vi "GDSIconEditor_CreateImageMask.vi"(1 "Flood Fill":bool, 2 "8-bit pixmap":u8[][](array[numeric])) -> (0 "Array":u8[](array[numeric]))   [LabVIEW 2020]
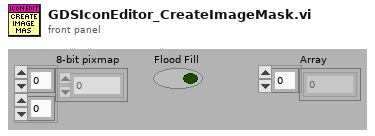
[diagram p1: front panel]
types:
  T1 = cluster{"disabled index (col)":i32, "disabled index (col)":i32}[]
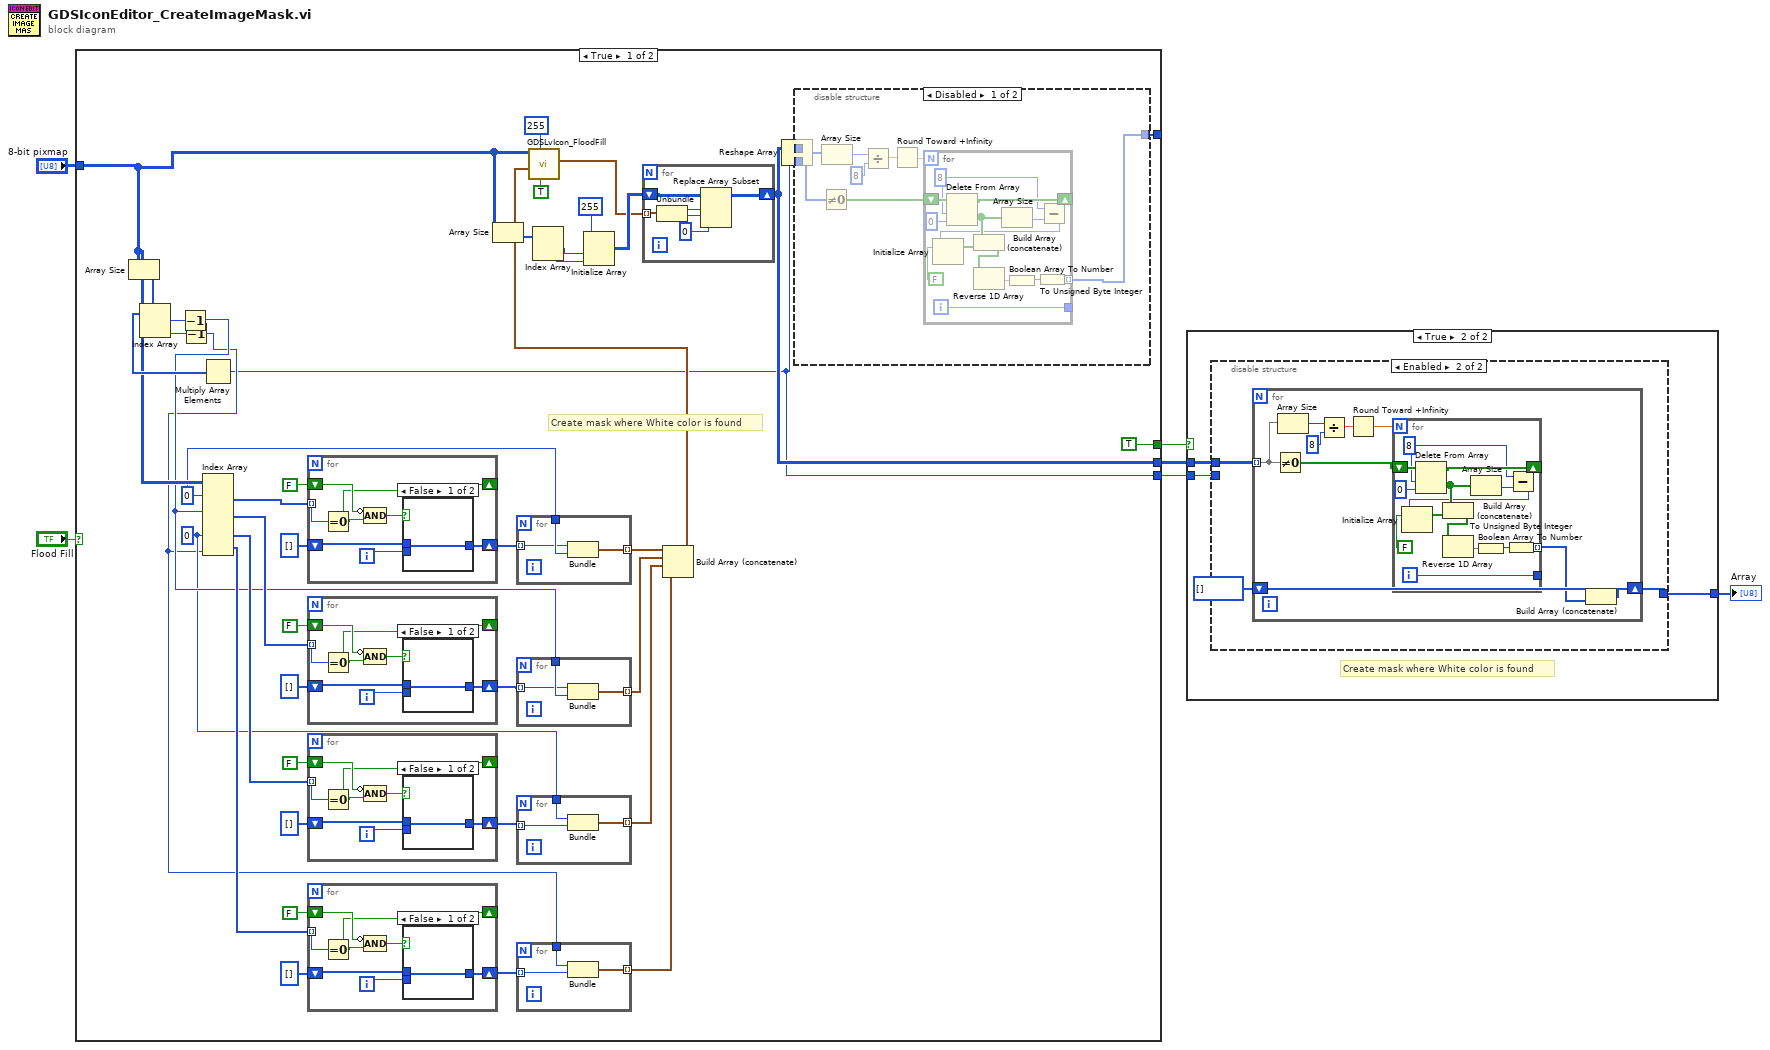
[diagram p0: block diagram]
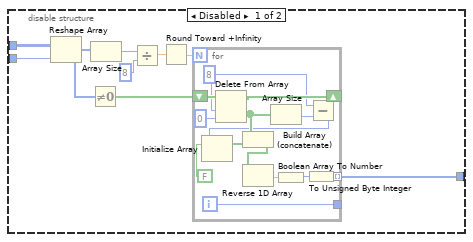
[diagram p3: hidden frame]
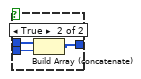
[diagram p5: hidden frame]
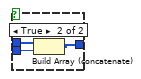
[diagram p6: hidden frame]
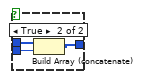
[diagram p7: hidden frame]
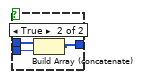
[diagram p8: hidden frame]
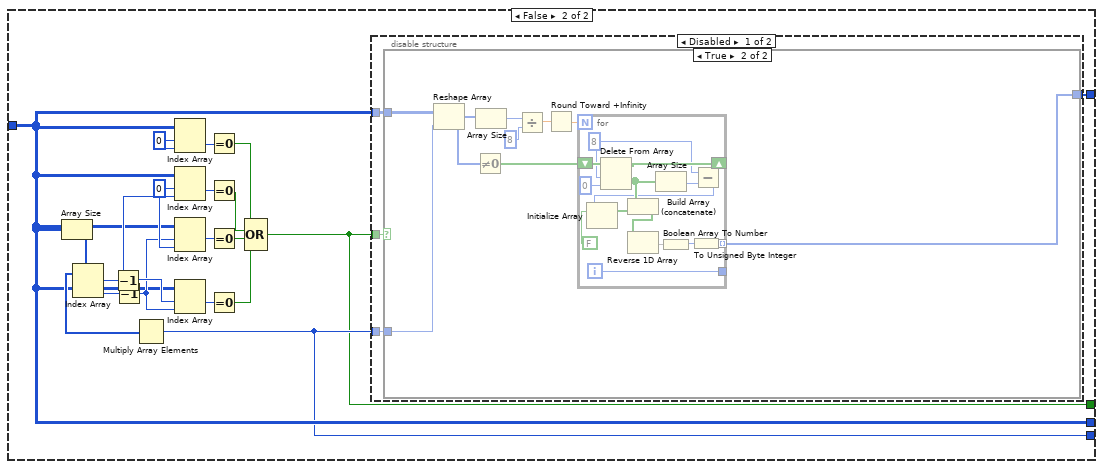
[diagram p9: hidden frame]
diagram:
  n1 = case shown="True" "Flood Fill" {
    tunnel: [w45 w144] -> _
    tunnel: "8-bit pixmap" -> [w43 w135]
    tunnel: [w9 w135] -> w4
    tunnel: [w8 w134] -> w3
    tunnel: [TRUE w133] -> w2
    frame True {
      w29 = 0 ("disabled index (col)")
      w25 = 0 ("disabled index (col)")
      # "Create mask where White color is found"
      n2 = Array Size(array=w43) -> (size(s)=w44:i32[])
      n3 = Index Array(array=w44) -> (element #1=w46:i32, element #2=w47:i32)  [unwired: 2 in]
      n4 = Decrement(x=w46) -> (x-1=w27:i32)
      n5 = Decrement(x=w47) -> (x-1=w23:i32)
      n6 = Multiply Array Elements(1:w44) -> (0:w8:i32)
      n7 = Index Array(array=w43, index (row) #1=w29, index (row) #2=w27, index (col) #3=w25, index (col) #4=w23) -> (element #1=w42:u8[], element #2=w37:u8[], element #3=w32:u8[], element #4=w31:u8[])  [unwired: 4 in]
      n8 = for {
        tunnel: w42 -> [w128] mode=indexing
        shift-right: [w125] -> _
        shift-left: FALSE -> [w127]
        shift-right: [w123] -> w30
        shift-left: i32[] [] -> [w124]
        i -> [w122]
        n9 = Equal To 0?(x=w128) -> (x = 0?=w125:bool)
        n10 = Compound Arithmetic op=AND(invert w127, w125) -> (w126:bool)
        n11 = case shown="False" w126 {
          tunnel: w124 -> [w129 w132]
          tunnel: [w129 w131] -> w123
          tunnel: w122 -> [_ w130]
          frame False {
          }
          frame True {
            n12 = Build Array (concatenate)(w132, w130) -> (w131:i32[])
          }
        }
      }
      n13 = for {
        tunnel: w37 -> [w117] mode=indexing
        shift-right: [w114] -> _
        shift-left: FALSE -> [w116]
        shift-right: [w112] -> w28
        shift-left: i32[] [] -> [w113]
        i -> [w111]
        n14 = Equal To 0?(x=w117) -> (x = 0?=w114:bool)
        n15 = Compound Arithmetic op=AND(invert w116, w114) -> (w115:bool)
        n16 = case shown="False" w115 {
          tunnel: w113 -> [w118 w121]
          tunnel: [w118 w120] -> w112
          tunnel: w111 -> [_ w119]
          frame False {
          }
          frame True {
            n17 = Build Array (concatenate)(w121, w119) -> (w120:i32[])
          }
        }
      }
      n18 = for {
        tunnel: w32 -> [w106] mode=indexing
        shift-right: [w103] -> _
        shift-left: FALSE -> [w105]
        shift-right: [w101] -> w26
        shift-left: i32[] [] -> [w102]
        i -> [w100]
        n19 = Equal To 0?(x=w106) -> (x = 0?=w103:bool)
        n20 = Compound Arithmetic op=AND(invert w105, w103) -> (w104:bool)
        n21 = case shown="False" w104 {
          tunnel: w102 -> [w107 w110]
          tunnel: [w107 w109] -> w101
          tunnel: w100 -> [_ w108]
          frame False {
          }
          frame True {
            n22 = Build Array (concatenate)(w110, w108) -> (w109:i32[])
          }
        }
      }
      n23 = for {
        tunnel: w31 -> [w95] mode=indexing
        shift-right: [w92] -> _
        shift-left: FALSE -> [w94]
        shift-right: [w90] -> w24
        shift-left: i32[] [] -> [w91]
        i -> [w89]
        n24 = Equal To 0?(x=w95) -> (x = 0?=w92:bool)
        n25 = Compound Arithmetic op=AND(invert w94, w92) -> (w93:bool)
        n26 = case shown="False" w93 {
          tunnel: w91 -> [w96 w99]
          tunnel: [w96 w98] -> w90
          tunnel: w89 -> [_ w97]
          frame False {
          }
          frame True {
            n27 = Build Array (concatenate)(w99, w97) -> (w98:i32[])
          }
        }
      }
      n28 = Array Size(array=w43) -> (size(s)=w15:i32[])
      n29 = for {
        tunnel: w30 -> [w87] mode=indexing
        tunnel: w29 -> [w88]
        tunnel: [w86] -> w22 mode=indexing
        n30 = Bundle(w87, "disabled index (col)"=w88) -> (w86:cluster{i32, "disabled index (col)":i32})  [unwired: 1 in]
      }
      n31 = for {
        tunnel: w28 -> [w84] mode=indexing
        tunnel: w27 -> [w85]
        tunnel: [w83] -> w21 mode=indexing
        n32 = Bundle(w84, w85) -> (w83:cluster{i32, i32})  [unwired: 1 in]
      }
      n33 = for {
        tunnel: w26 -> [w82] mode=indexing
        tunnel: w25 -> [w81]
        tunnel: [w80] -> w20 mode=indexing
        n34 = Bundle("disabled index (col)"=w81, w82) -> (w80:cluster{"disabled index (col)":i32, i32})  [unwired: 1 in]
      }
      n35 = for {
        tunnel: w24 -> [w79] mode=indexing
        tunnel: w23 -> [w78]
        tunnel: [w77] -> w19 mode=indexing
        n36 = Bundle(w78, w79) -> (w77:cluster{i32, i32})  [unwired: 1 in]
      }
      n37 = Index Array(array=w15) -> (element #1=w11:i32, element #2=w10:i32)  [unwired: 2 in]
      n38 = Initialize Array(u8 255 ("NewColor"), w11, w10) -> (w13:u8[][])
      n39 = Build Array (concatenate)(w22, w21, w20, w19) -> (w18:T1)
      n40 = call <resource>:"GDSLvIcon_FloodFill.vi"("4 (T) or 8 (F)"=TRUE, "NewColor"=u8 255, "StartPositions"=w18, "IconIn"=w43) -> ("PointsFilled"=w12:cluster{"y":i32, "x":i32}[])  [unwired: 5 in, 2 out]
      n41 = for {
        shift-right: [w71] -> w9
        shift-left: w13 -> [w76]
        tunnel: w12 -> [w75] mode=indexing
        n42 = Unbundle(w75) -> ("y"=w74:i32, "x"=w73:i32)
        n43 = Replace Array Subset(array=w76, new element=u8 0 ("new element/subarray"), index (row)=w74, index (col)=w73) -> (w71:u8[][])
      }
      n44 = disable-structure shown="Disabled" {
        disable-tunnel: [w56 _] -> w45
        disable-tunnel: w9 -> [w49 _]
        disable-tunnel: w8 -> [w48 _]
        frame Disabled {
          n45 = Reshape Array(w49, w48) -> (w55:u8[])
          n46 = Not Equal To 0?(x=w55) -> (x != 0?=w50:bool[])
          n47 = Array Size(array=w55) -> (size(s)=w54:i32)
          n48 = Divide(x=w54, y=8) -> (x/y=w52:dbl)
          n49 = Round Toward +Infinity(x=w52) -> (ceil(x): smallest int >= x=w51:dbl)
          n50 = for {
            N: w51 -> [_]
            shift-right: [w68] -> _
            shift-left: w50 -> [w70]
            tunnel: [w65] -> w56 mode=indexing
            tunnel: [w64] -> _
            i -> [w64]
            w59 = 8 ("length")
            n51 = Delete From Array(array=w70, length=w59, index=0) -> (deleted portion=w61:bool[], array with subset deleted=w68:bool[])
            n52 = Array Size(array=w61) -> (size(s)=w60:i32)
            n53 = Subtract(x=w59, y=w60) -> (x-y=w58:i32)
            n54 = Initialize Array(FALSE, w58) -> (w62:bool[])
            n55 = Build Array (concatenate)(w61, w62) -> (w63:bool[])
            n56 = Reverse 1D Array(array=w63) -> (reversed array=w66:bool[])
            n57 = Boolean Array To Number(Boolean array=w66) -> (number=w67:u32)
            n58 = To Unsigned Byte Integer(number=w67) -> (unsigned 8bit integer=w65:u8)
          }
        }
        frame Enabled {
        }
      }
    }
    frame False {
      w138 = 0 ("index (row)")
      w141 = 0 ("index (row)")
      n59 = Array Size(array=w135) -> (size(s)=w143:i32[])
      n60 = Index Array(array=w143) -> (element #1=w150:i32, element #2=w151:i32)  [unwired: 2 in]
      n61 = Decrement(x=w150) -> (x-1=w137:i32)
      n62 = Decrement(x=w151) -> (x-1=w136:i32)
      n63 = Multiply Array Elements(1:w143) -> (0:w134:i32)
      n64 = Index Array(array=w135, index (row)=w141, index (col)=w141) -> (element=w149:u8)
      n65 = Index Array(array=w135, index (row)=w138, index (col)=w137) -> (element=w148:u8)
      n66 = Index Array(array=w135, index (row)=w136, index (col)=w138) -> (element=w147:u8)
      n67 = Index Array(array=w135, index (row)=w137, index (col)=w136) -> (element=w146:u8)
      n68 = Equal To 0?(x=w149) -> (x = 0?=w142:bool)
      n69 = Equal To 0?(x=w148) -> (x = 0?=w140:bool)
      n70 = Equal To 0?(x=w147) -> (x = 0?=w139:bool)
      n71 = Equal To 0?(x=w146) -> (x = 0?=w145:bool)
      n72 = Compound Arithmetic op=OR(w142, w140, w139, w145) -> (w133:bool)
      n73 = disable-structure shown="Disabled" {
        disable-tunnel: [w155 _] -> w144
        disable-tunnel: w135 -> [w154 _]
        disable-tunnel: w134 -> [w153 _]
        disable-tunnel: w133 -> [w152 _]
        frame Disabled {
          n74 = case shown="True" w152 {
            tunnel: [_ w162] -> w155
            tunnel: w154 -> [_ w164]
            tunnel: w153 -> [_ w163]
            frame False {
            }
            frame True {
              n75 = Reshape Array(w164, w163) -> (w161:u8[])
              n76 = Not Equal To 0?(x=w161) -> (x != 0?=w156:bool[])
              n77 = Array Size(array=w161) -> (size(s)=w160:i32)
              n78 = Divide(x=w160, y=8) -> (x/y=w158:dbl)
              n79 = Round Toward +Infinity(x=w158) -> (ceil(x): smallest int >= x=w157:dbl)
              n80 = for {
                N: w157 -> [_]
                shift-right: [w176] -> _
                shift-left: w156 -> [w178]
                tunnel: [w173] -> w162 mode=indexing
                tunnel: [w172] -> _
                i -> [w172]
                w167 = 8 ("length")
                n81 = Delete From Array(array=w178, length=w167, index=0) -> (deleted portion=w169:bool[], array with subset deleted=w176:bool[])
                n82 = Array Size(array=w169) -> (size(s)=w168:i32)
                n83 = Subtract(x=w167, y=w168) -> (x-y=w166:i32)
                n84 = Initialize Array(FALSE, w166) -> (w170:bool[])
                n85 = Build Array (concatenate)(w169, w170) -> (w171:bool[])
                n86 = Reverse 1D Array(array=w171) -> (reversed array=w174:bool[])
                n87 = Boolean Array To Number(Boolean array=w174) -> (number=w175:u32)
                n88 = To Unsigned Byte Integer(number=w175) -> (unsigned 8bit integer=w173:u8)
              }
            }
          }
        }
        frame Enabled {
        }
      }
    }
  }
  n89 = case shown="True" w2 {
    tunnel: w4 -> [_ w181]
    tunnel: w3 -> [_ w180]
    tunnel: [_ w179] -> w1
    frame False {
    }
    frame True {
      # "Create mask where White color is found"
      n90 = disable-structure shown="Enabled" {
        disable-tunnel: w181 -> [w184 w207]
        disable-tunnel: w180 -> [w183 _]
        disable-tunnel: [w182 w205] -> w179
        frame Disabled {
          n91 = Reshape Array(w184, w183) -> (w185:u8[])
          n92 = Not Equal To 0?(x=w185) -> (x != 0?=w190:bool[])
          n93 = Array Size(array=w185) -> (size(s)=w186:i32)
          n94 = Divide(x=w186, y=8) -> (x/y=w188:dbl)
          n95 = Round Toward +Infinity(x=w188) -> (ceil(x): smallest int >= x=w189:dbl)
          n96 = for {
            N: w189 -> [_]
            shift-right: [w202] -> _
            shift-left: w190 -> [w204]
            tunnel: [w199] -> w182 mode=indexing
            tunnel: [w198] -> _
            i -> [w198]
            w193 = 8 ("length")
            n97 = Delete From Array(array=w204, length=w193, index=0) -> (deleted portion=w195:bool[], array with subset deleted=w202:bool[])
            n98 = Array Size(array=w195) -> (size(s)=w194:i32)
            n99 = Subtract(x=w193, y=w194) -> (x-y=w192:i32)
            n100 = Initialize Array(FALSE, w192) -> (w196:bool[])
            n101 = Build Array (concatenate)(w195, w196) -> (w197:bool[])
            n102 = Reverse 1D Array(array=w197) -> (reversed array=w200:bool[])
            n103 = Boolean Array To Number(Boolean array=w200) -> (number=w201:u32)
            n104 = To Unsigned Byte Integer(number=w201) -> (unsigned 8bit integer=w199:u8)
          }
        }
        frame Enabled {
          n105 = for {
            tunnel: w207 -> [w213] mode=indexing
            shift-right: [w208] -> w205
            shift-left: u8[] [] -> [w210]
            n106 = Not Equal To 0?(x=w213) -> (x != 0?=w211:bool[])
            n107 = Array Size(array=w213) -> (size(s)=w214:i32)
            n108 = Divide(x=w214, y=8) -> (x/y=w216:dbl)
            n109 = Round Toward +Infinity(x=w216) -> (ceil(x): smallest int >= x=w212:dbl)
            n110 = for {
              N: w212 -> [_]
              shift-right: [w228] -> _
              shift-left: w211 -> [w230]
              tunnel: [w225] -> w209 mode=indexing
              tunnel: [w224] -> _
              i -> [w224]
              w219 = 8 ("length")
              n111 = Delete From Array(array=w230, length=w219, index=0) -> (deleted portion=w221:bool[], array with subset deleted=w228:bool[])
              n112 = Array Size(array=w221) -> (size(s)=w220:i32)
              n113 = Subtract(x=w219, y=w220) -> (x-y=w218:i32)
              n114 = Initialize Array(FALSE, w218) -> (w222:bool[])
              n115 = Build Array (concatenate)(w221, w222) -> (w223:bool[])
              n116 = Reverse 1D Array(array=w223) -> (reversed array=w226:bool[])
              n117 = Boolean Array To Number(Boolean array=w226) -> (number=w227:u32)
              n118 = To Unsigned Byte Integer(number=w227) -> (unsigned 8bit integer=w225:u8)
            }
            n119 = Build Array (concatenate)(w210, w209) -> (w208:u8[])
          }
        }
      }
    }
  }
  "Array" <- w1
